vi "DAQ mx Channel Listing.vi"() -> ()   [LabVIEW 2021, in "Safety Release Test VI's.lvlib"]
uses:
  Safety Release Test VI's.lvlib
  Main Engine/Controls/Main Engine Hardware Info Data Cluster.ctl
  Main Engine/Controls/Main Engine DAQ Device Info.ctl
  <vilib>/nisyscfg/nisyscfg.lvlib
  <resource>/objmgr/nicriosae.rc
  <resource>/objmgr/daqmx.rc
panel:
  out "Array 2":string[](array[string])
  out "Array":u32[](array[numeric])
  out "Resources out":refnum<k20>[](array[refnum])
  out "CPU Session":refnum<k21>
  out "DAQ Device Info":T1[](array[typedef])
  out "Hardware Info":T2[](array[typedef]) {"Is Present?" items=["Initializing"=-2, "Unknown"=-1, "Not Present"=0, "Present"=1]}
  out "error out":errorcluster
  in  "error in":errorcluster
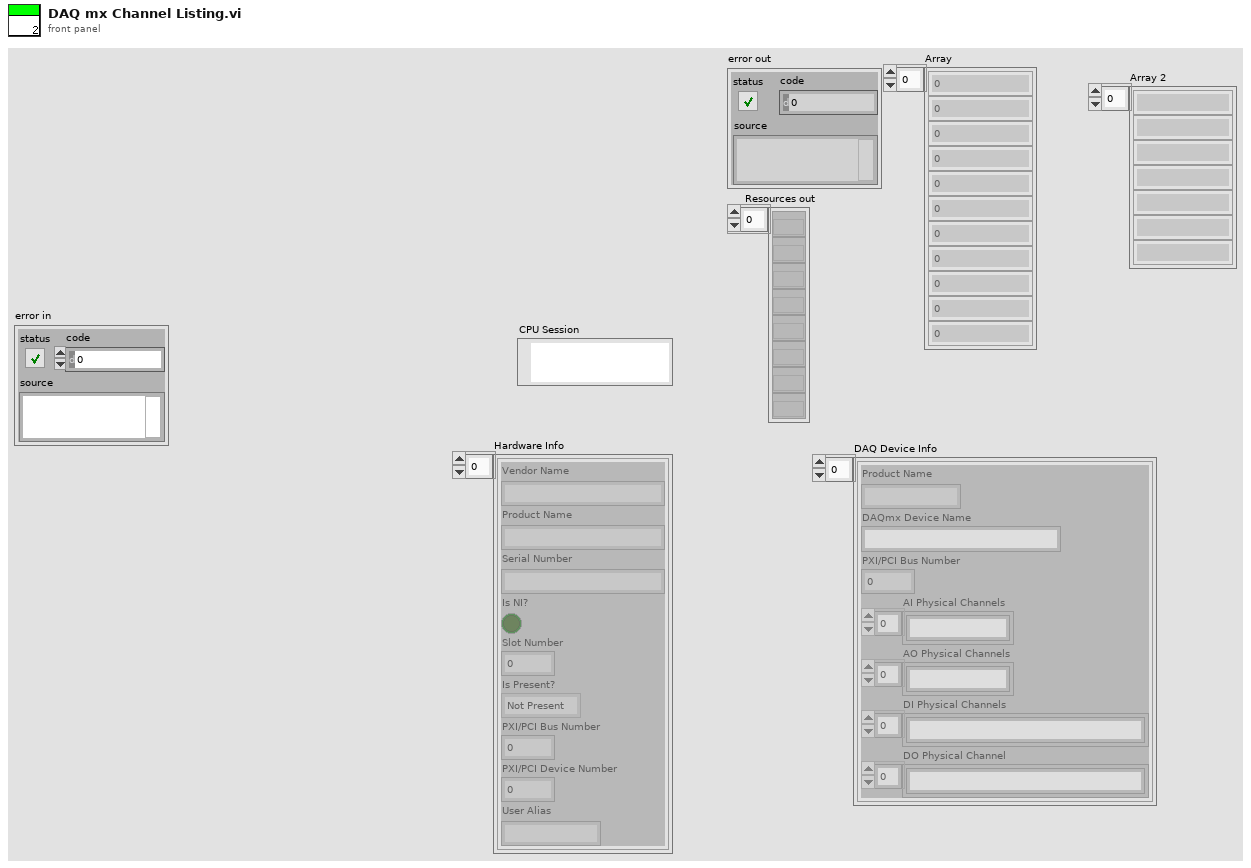
[diagram p1: front panel]
types:
  T1 = typedef "Main Engine DAQ Device Info.ctl" = cluster{"Product Name":string, "DAQmx Device Name":string, "PXI/PCI Bus Number":u32, "AI Physical Channels":string[], "AO Physical Channels":string[], "DI Physical Channels":string[], "DO Physical Channel":string[]}
  T2 = typedef "Main Engine Hardware Info Data Cluster.ctl" = cluster{"Vendor Name":string, "Product Name":string, "Serial Number":string, "Is NI?":bool, "Slot Number":i32, "Is Present?":i32, "PXI/PCI Bus Number":u32, "PXI/PCI Device Number":u32, "User Alias":string}
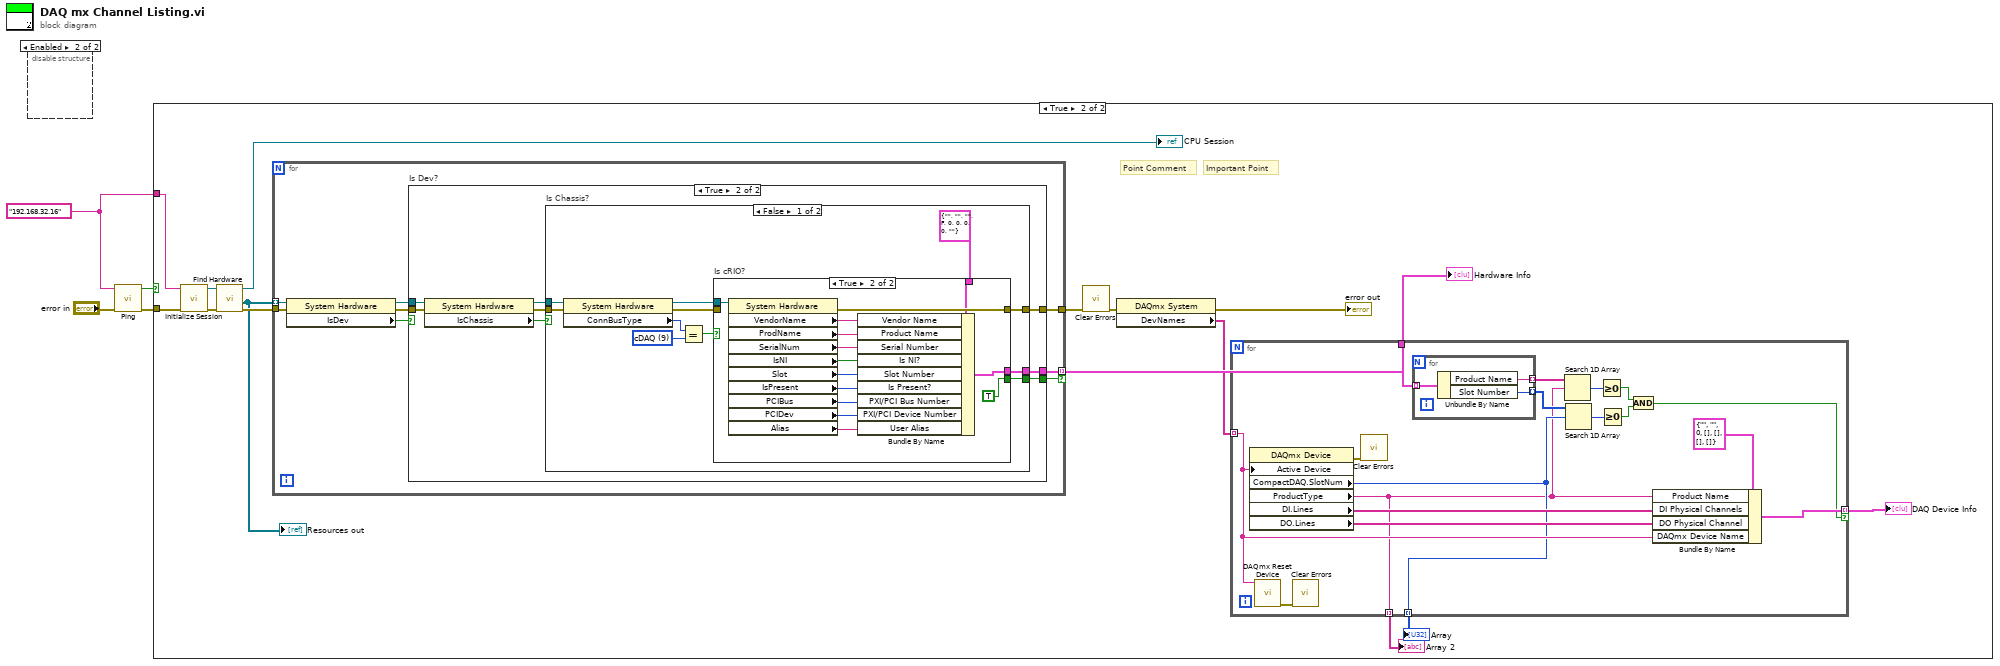
[diagram p0: block diagram]
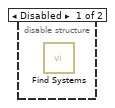
[diagram p6: hidden frame]
diagram:
  w3 = "192.168.32.16" ("hostNameOrAddress")
  n1 = disable-structure shown="Enabled" {
    frame Disabled {
      n2 = call <vilib>:"Find Systems.vi"() -> ()  [unwired: 9 in, 3 out]
    }
    frame Enabled {
    }
  }
  n3 = call "Ping.vi"("error in"="error in", "hostNameOrAddress"=w3) -> ("error out"=w2:errorcluster, "Ping Status"=w1:bool)  [unwired: 8 in]
  n4 = case shown="True" w1 {
    tunnel: w3 -> [_ w16]
    tunnel: w2 -> [_ w11]
    frame False {
    }
    frame True {
      # "Important Point"
      # "Point Comment"
      n5 = call <vilib>:"Initialize Session.vi"("error in (no error)"=w11, "Target (localhost)"=w16) -> ("error out"=w9:errorcluster, "Session out"=w10:refnum<k21>)  [unwired: 8 in]
      n6 = call <vilib>:"Find Hardware.vi"("error in (no error)"=w9, "Session in"=w10) -> ("error out"=w15:errorcluster, "Resources out"=w8:refnum<k20>[], "Session out"=→"CPU Session":refnum<k21>)  [unwired: 6 in, 1 out]
      "Resources out" <- w8
      n7 = for {
        tunnel: w8 -> [w47] mode=indexing
        tunnel: w15 -> [w43]
        tunnel: [w42] -> w14
        tunnel: [w41] -> w19 mode=indexing if=w40
        n8 = property class="System Hardware"(reference=w47, error in=w43) -> (reference out=w46:refnum<k20>, error out=w45:errorcluster, "IsDev"=w44:bool)
        n9 = case "Is Dev?" shown="True" w44 {
          tunnel: w46 -> [_ w56]
          tunnel: w45 -> [w48 w55]
          tunnel: [w48 w51] -> w42
          tunnel: [_ w50] -> w40
          tunnel: [_ w49] -> w41
          frame False {
          }
          frame True {
            n10 = property class="System Hardware"(reference=w56, error in=w55) -> (reference out=w54:refnum<k20>, error out=w52:errorcluster, "IsChassis"=w53:bool)
            n11 = case "Is Chassis?" shown="False" w53 {
              tunnel: w54 -> [w67 _]
              tunnel: w52 -> [w66 w83]
              tunnel: [w61 w83] -> w51
              tunnel: [w59 _] -> w50
              tunnel: [w58 _] -> w49
              frame False {
                w64 = u32 9 items=["BuiltIn/System", "PXI/PCI", "USB", "GPIB", "VXI", "Serial", "TCP/IP", "cRIO", "SCXI", "cDAQ", "SwitchBlock", "SCC", "FireWire", "Accessory", "CAN", "SwitchBlock Device"] ("Devices & Chassis:Connects To Bus Type")
                n12 = property class="System Hardware"(reference=w67, error in=w66) -> (reference out=w60:refnum<k20>, error out=w62:errorcluster, "ConnBusType"=w65:u32)
                n13 = Equal?(x=w65, y=w64) -> (x = y?=w63:bool)
                n14 = case "Is cRIO?" shown="True" w63 {
                  tunnel: w62 -> [w68 _]
                  tunnel: [w68 w82] -> w61
                  tunnel: w60 -> [_ w71]
                  tunnel: [_ TRUE] -> w59
                  tunnel: [_ w75] -> w58
                  tunnel: T2 {"Vendor Name"="", "Product Name"="", "Serial Number"="", "Is NI?"=FALSE, "Slot Number"=0, "Is Present?"=0, "PXI/PCI Bus Number"=0, "PXI/PCI Device Number"=0, "User Alias"=""} ("Hardware Info") -> [_ w70]
                  frame False {
                  }
                  frame True {
                    n15 = property class="System Hardware"(reference=w71) -> (error out=w82:errorcluster, "VendorName"=w76:string, "ProdName"=w77:string, "SerialNum"=w78:string, "IsNI"=w79:bool, "Slot"=w72:i32, "IsPresent"=w80:i32, "PCIBus"=w74:u32, "PCIDev"=w73:u32, "Alias"=w69:string)  [unwired: 1 in, 1 out]
                    n16 = Bundle By Name(cluster=w70, "Vendor Name"=w76, "Product Name"=w77, "Serial Number"=w78, "Is NI?"=w79, "Slot Number"=w72, "Is Present?"=w80, "PXI/PCI Bus Number"=w74, "PXI/PCI Device Number"=w73, "User Alias"=w69) -> (w75:T2)
                  }
                }
              }
              frame True {
              }
            }
          }
        }
      }
      "Hardware Info" <- w19
      n17 = call <vilib>:"Clear Errors.vi"("error in (no error)"=w14) -> ("error out"=w12:errorcluster)  [unwired: 5 in, 1 out]
      n18 = property class="DAQmx System"(error in=w12) -> (error out=→"error out":errorcluster, "DevNames"=w13:tag[])  [unwired: 1 in, 1 out]
      n19 = for {
        tunnel: w13 -> [w30] mode=indexing
        tunnel: w19 -> [w36]
        tunnel: [w35] -> w18 mode=indexing if=w22
        tunnel: [w27] -> w6 mode=indexing
        tunnel: [w20] -> w5 mode=indexing
        n20 = property class="DAQmx Device"("Active Device"=w30) -> (error out=w32:errorcluster, "CompactDAQ.SlotNum"=w27:u32, "ProductType"=w20:string, "DI.Lines"=w34:tag[], "DO.Lines"=w33:tag[])  [unwired: 2 in, 1 out]
        n21 = call <vilib>:"DAQmx Reset Device.vi"("device in"=w30) -> ("error out"=w31:errorcluster)  [unwired: 14 in]
        n22 = call <vilib>:"Clear Errors.vi"("error in (no error)"=w31) -> ()  [unwired: 5 in, 2 out]
        n23 = call <vilib>:"Clear Errors.vi"("error in (no error)"=w32) -> ()  [unwired: 5 in, 2 out]
        n24 = for {
          tunnel: w36 -> [w39] mode=indexing
          tunnel: [w38] -> w29 mode=indexing
          tunnel: [w37] -> w28 mode=indexing
          n25 = Unbundle By Name(w39) -> ("Product Name"=w38:string, "Slot Number"=w37:i32)
        }
        n26 = Search 1D Array(1D array=w29, element=w20) -> (index of element=w26:i32)  [unwired: 1 in]
        n27 = Search 1D Array(1D array=w28, element=w27) -> (index of element=w25:i32)  [unwired: 1 in]
        n28 = Greater Or Equal To 0?(x=w26) -> (x >= 0?=w24:bool)
        n29 = Greater Or Equal To 0?(x=w25) -> (x >= 0?=w23:bool)
        n30 = And(x=w24, y=w23) -> (x .and. y?=w22:bool)
        n31 = Bundle By Name(cluster=T1 {"Product Name"="", "DAQmx Device Name"="", "PXI/PCI Bus Number"=0, "AI Physical Channels"=[], "AO Physical Channels"=[], "DI Physical Channels"=[], "DO Physical Channel"=[]} ("Daq Device Info"), "Product Name"=w20, "DI Physical Channels"=w34, "DO Physical Channel"=w33, "DAQmx Device Name"=w30) -> (w35:T1)
      }
      "DAQ Device Info" <- w18
      "Array" <- w6
      "Array 2" <- w5
    }
  }
